vi "Initialize.vi"(0 "Staff Manager Model in":refnum<class "Staff Manager Model.lvclass">, 11 "error in (no error)":errorcluster) -> (4 "Staff Manager Model out":refnum<class "Staff Manager Model.lvclass">, 15 "error out":errorcluster)   [LabVIEW 2023, in "Staff Manager Model.lvlib" / "Staff Manager Model.lvclass"]
uses:
  Staff Manager Model.lvclass
  Staff Manager Model.lvclass/Staff Manager Model.ctl
  <vilib>/ActorFramework/Actor/Actor.lvclass
  C:/Users/bhaghyaraj/Trainings/NI Actor Framework/SDLC/Model Base/Model Base/Model Base.lvclass
  C:/Program Files/National Instruments/LabVIEW 2023/vi.lib/ActorFramework/Actor/Actor.lvclass
  C:/Users/bhaghyaraj/Trainings/NI Actor Framework/SDLC/Interfaces/Model Base/Incoming Model Base Interface.lvclass
  C:/Users/bhaghyaraj/Trainings/NI Actor Framework/SDLC/Staff Manager Model/Staff Manager Model/Staff Manager Model.lvclass
  Staff Manager UI/Staff Manager UI/Staff Manager UI.lvclass
  C:/Users/bhaghyaraj/Trainings/NI Actor Framework/SDLC/UI Base/UI Base/UI Base.lvclass
  C:/Users/bhaghyaraj/Trainings/NI Actor Framework/SDLC/Staff Manager UI/Staff Manager UI/Staff Manager UI.lvclass
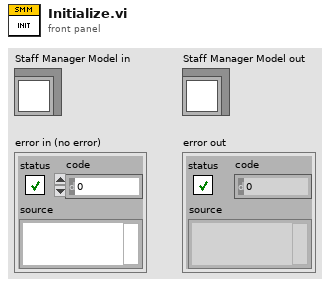
[diagram p1: front panel]
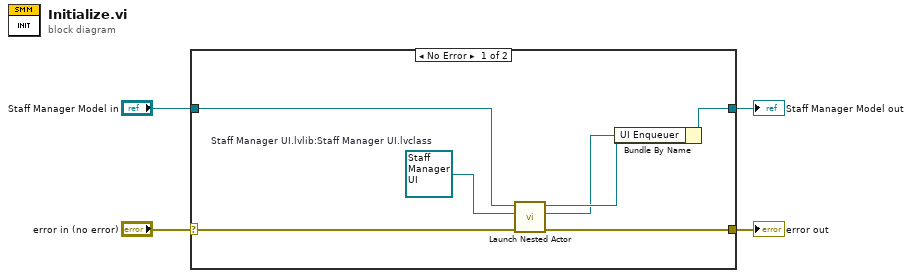
[diagram p0: block diagram]
diagram:
  n1 = case shown="No Error" "error in (no error)" {
    selector: "error in (no error)" -> [w11 w13]
    tunnel: [w10 w13] -> w3
    tunnel: [w7 w12] -> w1
    tunnel: "Staff Manager Model in" -> [w8 w12]
    frame No Error {
      w5 = refnum<class "Staff Manager UI.lvclass"> refnum  # Staff Manager UI.lvlib:Staff Manager UI.lvclass
      n2 = call <vilib>:"Launch Nested Actor.vi"("error in (no error)"=w11, "Nested Actor"=w5, "Caller Actor in"=w8) -> ("error out"=w10:errorcluster, "Nested Actor's Enqueuer"=w6:refnum<class "Message Enqueuer.lvclass">, "Caller Actor out"=w9:refnum<class "Staff Manager Model.lvclass">)  [unwired: 6 in]
      n3 = Bundle By Name(cluster=w9, "UI Enqueuer"=w6) -> (w7:refnum<class "Staff Manager Model.lvclass">)
    }
    frame Error {
    }
  }
  "error out" <- w3
  "Staff Manager Model out" <- w1
